vi "CreateVisitor.vi"(4 "Agents class path":path, 6 "Controls Cluster":T1(array[cluster]), 7 "Library Basepath":path, 8 "error in":errorcluster, 9 "Agents VI Path":path, 10 "VI Name":string, 11 "Class Name":string) -> (0 "error out":errorcluster, 2 "Visitor Class Path":path)   [LabVIEW 2009, in "HGF_VisitorGenerator.lvlib"]
doc: "create single visitor class and its member VIs to execute one of the agents public VI interfaces"
uses:
  HGF_VisitorGenerator.lvlib
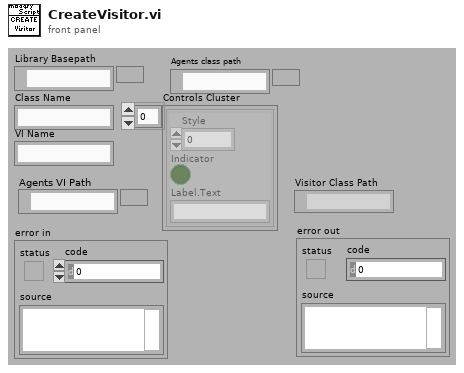
[diagram p1: front panel]
types:
  T1 = cluster{"Style":u32, "Indicator":bool, "Label.Text":string}[]
  T2 = enum32{"invalid scope", "public", "private", "protected", "community"}
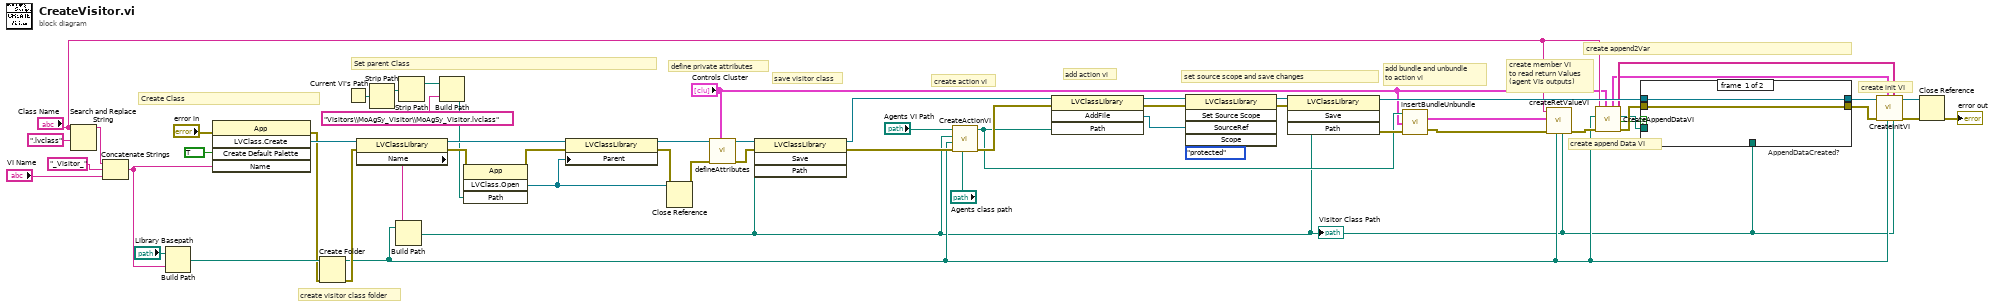
[diagram p0: block diagram]
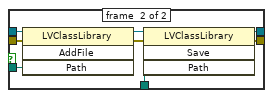
[diagram p2: hidden frame]
diagram:
  # "create init VI"
  # "create append Data VI"
  # "create member VI\nto read return Values\n(agent VIs outputs)"
  # "create append2Var"
  # "add bundle and unbundle\nto action vi"
  # "define private attributes"
  # "set source scope and save changes"
  # "add action vi"
  # "create action vi"
  # "create visitor class folder"
  # "save visitor class"
  # "Set parent Class"
  # "Create Class"
  n1 = Search and Replace String(input string="Class Name", search string=".lvclass") -> (result string=w56:string)  [unwired: 6 in, 3 out]
  n2 = Concatenate Strings(w56, "_Visitor_" ("string"), "VI Name") -> (w52:string)
  n3 = Build Path(base path="Library Basepath", name or relative path=w52) -> (appended path=w48:path)
  n4 = invoke class="App" method="LVClass.Create"(error in="error in", "Create Default Palette"=TRUE ("Create:Default Palette"), "Name"=w52) -> (error out=w44:errorcluster, "LVClass.Create"=w50:refnum<vi>)  [unwired: 2 in, 3 out]
  n5 = Create Folder(path (use dialog)=w48, error in=w44) -> (created path=w8:path, error out=w40:errorcluster)  [unwired: 1 in, 1 out]
  n6 = Current VI's Path() -> (path=w5:path)
  n7 = property class="LVClassLibrary"(reference=w50, error in=w40) -> (reference out=w41:refnum<vi>, error out=w42:errorcluster, "Name"=w49:string)
  n8 = Strip Path(path=w5) -> (stripped path=w4:path)  [unwired: 1 out]
  n9 = Build Path(base path=w8, name or relative path=w49) -> (appended path=w7:path)
  "Visitor Class Path" <- w7
  n10 = Strip Path(path=w4) -> (stripped path=w3:path)  [unwired: 1 out]
  n11 = Build Path(base path=w3, name or relative path="Visitors\\MoAgSy_Visitor\\MoAgSy_Visitor.lvclass") -> (appended path=w1:path)
  n12 = invoke class="App" method="LVClass.Open"(error in=w42, "Path"=w1) -> (error out=w43:errorcluster, "LVClass.Open"=w39:refnum<vi>)  [unwired: 2 in, 2 out]
  n13 = property class="LVClassLibrary"(reference=w41, error in=w43, "Parent"=w39) -> (reference out=w30:refnum<vi>, error out=w38:errorcluster)
  n14 = Close Reference(reference=w39, error in (no error)=w38) -> (error out=w28:errorcluster)
  n15 = call "defineAttributes.vi"("Controls Cluster"="Controls Cluster", "error in (no error)"=w28, "Class Reference"=w30) -> ("error out"=w27:errorcluster, "Class Reference out"=w29:refnum<vi>)  [unwired: 7 in]
  n16 = invoke class="LVClassLibrary" method="Save"(reference=w29, error in=w27, "Path"=w7) -> (reference out=w47:refnum<vi>, error out=w26:errorcluster)  [unwired: 1 in, 2 out]
  n17 = call "CreateActionVI.vi"("Agents class path"="Agents class path", "error in"=w26, "VisitorFolder"=w8, "VisitorClassPath"=w7, "AgentsPublic"="Agents VI Path") -> ("error out"=w46:errorcluster, "actionVIPath"=w23:path)  [unwired: 5 in]
  n18 = invoke class="LVClassLibrary" method="AddFile"(reference=w47, error in=w46, "Path"=w23) -> (reference out=w37:refnum<vi>, error out=w35:errorcluster, "AddFile"=w33:refnum<vi>)  [unwired: 1 in, 1 out]
  n19 = invoke class="LVClassLibrary" method="Set Source Scope"(reference=w37, error in=w35, "SourceRef"=w33, "Scope"=T2."protected" ("scope")) -> (reference out=w36:refnum<vi>, error out=w32:errorcluster)  [unwired: 1 in, 3 out]
  n20 = invoke class="LVClassLibrary" method="Save"(reference=w36, error in=w32, "Path"=w7) -> (reference out=w21:refnum<vi>, error out=w24:errorcluster)  [unwired: 1 in, 2 out]
  n21 = call "insertBundleUnbundle.vi"("error in (no error)"=w24, "Controls Cluster"="Controls Cluster", "action vi path"=w23) -> ("error out"=w12:errorcluster, "Indicators"=w10:cluster{"Style":u32, "Label.Text":string, i32}[])
  n22 = call "createRetValueVI.vi"("visitor class path"=w7, "visitor base path"=w8, "error in (no error)"=w12, "Indicators"=w10, "Class Name"="Class Name") -> ("error out"=w11:errorcluster)  [unwired: 6 in]
  n23 = call "CreateAppendDataVI.vi"("Controls Cluster"="Controls Cluster", "error in (no error)"=w11, "Visitor base path"=w8, "Classname"="Class Name") -> ("error out"=w22:errorcluster, "AppendDataVI created"=w19:bool, "Append Data Path"=w20:path, "VariantAttNames"=w14:string[], "controls"=w13:cluster{"Style":u32, "Label.Text":string, i32}[])  [unwired: 3 in]
  n24 = case "AppendDataCreated?" shown="True" w19 {
    tunnel: [w60 w68] -> w17
    tunnel: [w59 w67] -> w15
    tunnel: w7 -> [_ w66]
    tunnel: w22 -> [w59 w65]
    tunnel: w21 -> [w60 w63]
    tunnel: w20 -> [_ w61]
    frame #0 {
    }
    frame #1 {
      n25 = invoke class="LVClassLibrary" method="AddFile"(reference=w63, error in=w65, "Path"=w61) -> (reference out=w62:refnum<vi>, error out=w64:errorcluster)  [unwired: 1 in, 2 out]
      n26 = invoke class="LVClassLibrary" method="Save"(reference=w62, error in=w64, "Path"=w66) -> (reference out=w68:refnum<vi>, error out=w67:errorcluster)  [unwired: 1 in, 2 out]
    }
  }
  n27 = call "CreateInitVI.vi"("visitor class path"=w7, "VariantAttNames"=w14, "visitor base path"=w8, "controls"=w13, "error in (no error)"=w15, "Class Reference"=w17) -> ("error out"=w16:errorcluster, "dup Class Reference"=w18:refnum<vi>)  [unwired: 4 in]
  n28 = Close Reference(reference=w18, error in (no error)=w16) -> (error out=→"error out":errorcluster)
